vi "JogVertical.vi"(11 "Numeric":dbl) -> ()   [LabVIEW 2020]
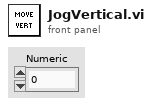
[diagram p1: front panel]
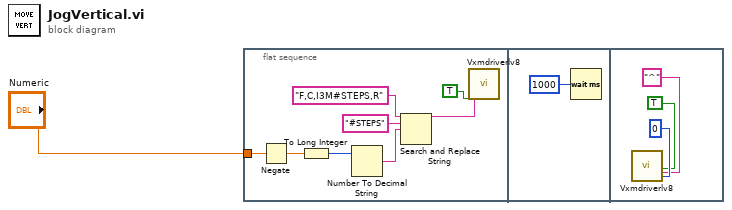
[diagram p0: block diagram]
diagram:
  n1 = flat-sequence {
    tunnel: "Numeric" -> [w2]
    frame #0 {
      n2 = Negate(x=w2) -> (-x=w3:dbl)
      n3 = To Long Integer(number=w3) -> (32bit integer=w4:i32)
      n4 = Number To Decimal String(number=w4) -> (decimal integer string=w9:string)  [unwired: 1 in]
      n5 = Search and Replace String(input string="F,C,I3M#STEPS,R" ("Chars to send"), search string="#STEPS", replace string=w9) -> (result string=w8:string)  [unwired: 5 in, 3 out]
      n6 = call "Vxmdriverlv8.Vi"("Send\nchars\nto port"=TRUE, "Chars to send"=w8) -> ()  [unwired: 20 in, 6 out]
    }
    frame #1 {
      n7 = Wait (ms)(milliseconds to wait=u32 1000) -> ()  [unwired: 1 out]
    }
    frame #2 {
      n8 = call "Vxmdriverlv8.Vi"("Wait\nfor \nchar"=TRUE, "Char(s) to wait for"="^", "Char\nTimeout\nTime (ms)"=0) -> ()  [unwired: 19 in, 6 out]
    }
  }
